vi "Post processing inversion hatch detector.vi"(7 "error in":errorcluster) -> (27 "error out":errorcluster)   [LabVIEW 2018]
uses:
  <vilib>/vision/NI_Vision_Development_Module.lvlib
panel:
  out "Particle Reports (Pixels)":T1(array[cluster]) {"Orientation" format="%.2f"; "Dimensions"."Height" format="%.2f"; "Dimensions"."Width" format="%.2f"; "Center of Mass"."Y" format="%.2f"; "Center of Mass"."X" format="%.2f"; "Bounding Rect"."Bottom" format="%.2f"; "Bounding Rect"."Right" format="%.2f"; "Bounding Rect"."Top" format="%.2f"; "Bounding Rect"."Left" format="%.2f"; "Number of Holes" format="%.2f"; "Area" format="%.2f"}
  out "Image Out 2":T2(plugin-control)
  in  "error in 2":errorcluster
  out "Image Out":T2(plugin-control)
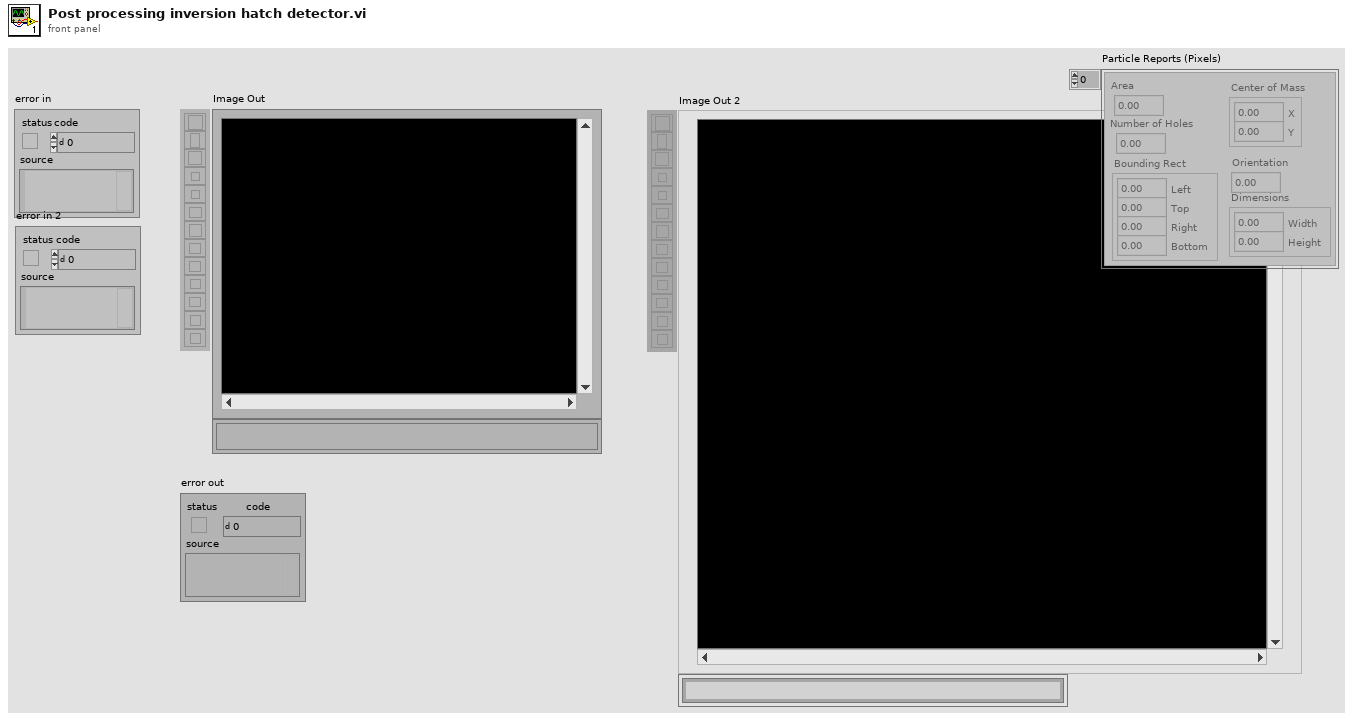
[diagram p1: front panel]
types:
  T1 = cluster{"Area":dbl, "Number of Holes":dbl, "Bounding Rect":cluster{"Left":dbl, "Top":dbl, "Right":dbl, "Bottom":dbl}, "Center of Mass":cluster{"X":dbl, "Y":dbl}, "Orientation":dbl, "Dimensions":cluster{"Width":dbl, "Height":dbl}}[]
  T2 = typedef "IMAQ Image.ctl" = refnum<image>
  T3 = cluster{"Desired Font (Application)":enum16{"User-specified Font", "Application Font", "System Font", "Dialog Font"}, "[User-specified Font]":cluster{"Font Name":string, "Size":i16, "Strikeout?":bool, "Italic?":bool, "Underline?":bool, "Outline?":bool, "Shadow?":bool, "Bold?":bool, "Rotation Angle":dbl}, "Horizontal Alignment":i16, "Vertical Alignment":i16}
  T4 = typedef "Image Type" = u32
  T5 = cluster{"Measurement Parameter":i32, "Range Lower Value":dbl, "Range Upper Value":dbl, "Range":bool, "Measurement Type":bool}[]
  T6 = cluster{"Area":dbl, "Number of Holes":dbl, "Bounding Rect":cluster{"Left":dbl, "Top":dbl, "Right":dbl, "Bottom":dbl}, "Center of Mass":cluster{"X":dbl, "Y":dbl}, "Orientation":dbl, "Dimensions":cluster{"Width":dbl, "Height":dbl}}
  T7 = cluster{"Left":dbl, "Top":dbl, "Right":dbl, "Bottom":dbl}
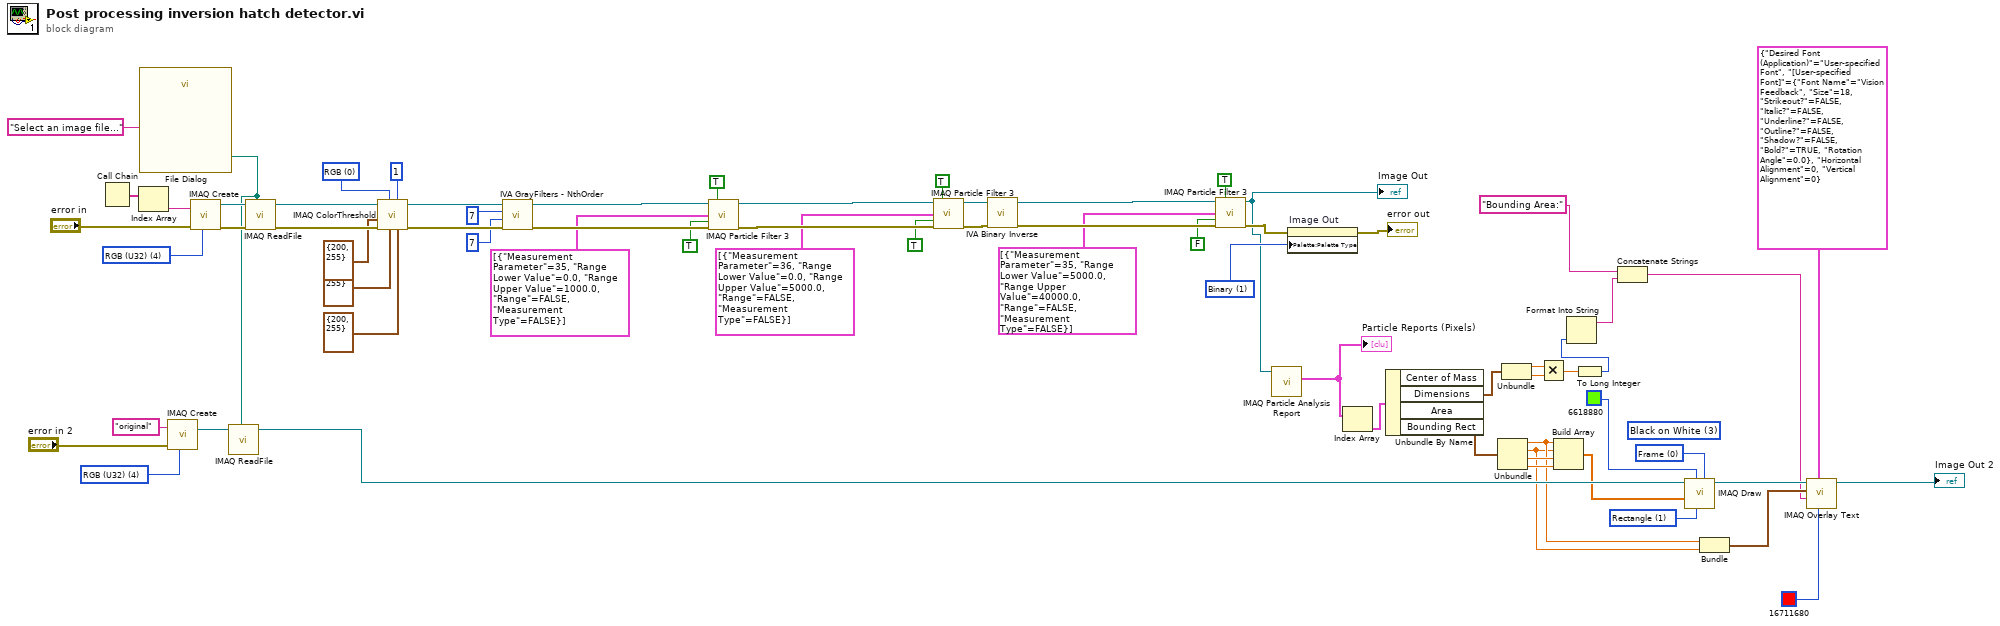
[diagram p0: block diagram]
diagram:
  (unwired) 3 items=["White", "Black", "Inverted", "Black on White", "White on Black"] ("Color")
  w21 = u16 1 items=["Line", "Rectangle", "Oval"] ("Shape to draw")
  w22 = u16 0 items=["Frame", "Paint", "Invert Frame", "Invert Paint"] ("Draw Mode")
  w31 = T4 4 items=["Grayscale (U8)", "Grayscale (I16)", "Grayscale (SGL)", "Complex (CSG)", "RGB (U32)", "HSL (U32)", "RGB (U64)", "Grayscale (U16)"] ("Image Type")
  w32 = u32 1 items=["Grayscale", "Binary", "Gradient", "Rainbow", "Temperature", "User Defined", "Binary 16 Bit", "Gradient 16 Bit", "Rainbow 16 Bit", "Temperature 16 Bit", "User Defined 16 Bit"] ("Palette Type")
  w60 = u16 0 items=["RGB", "HSL", "HSV", "HSI"] ("Color Mode")
  w62 = T4 4 items=["Grayscale (U8)", "Grayscale (I16)", "Grayscale (SGL)", "Complex (CSG)", "RGB (U32)", "HSL (U32)", "RGB (U64)", "Grayscale (U16)"] ("Image Type")
  n1 = Call Chain() -> (call chain=w65:string[])
  n2 = Index Array(array=w65) -> (element=w64:string)  [unwired: 1 in]
  n3 = call "File Dialog"("prompt"="Select an image file...") -> ("selected path"=w27:path)  [unwired: 6 in, 8 out]
  n4 = call "IMAQ Create"("Image Name"="original", "Image Type"=w31, "error in (no error)"="error in 2") -> ("New Image"=w28:T2)  [unwired: 1 in, 2 out]
  n5 = call "IMAQ Create"("Image Name"=w64, "Image Type"=w62, "error in (no error)"="error in") -> ("New Image"=w68:T2, "error out"=w67:errorcluster)  [unwired: 1 in, 1 out]
  n6 = call "IMAQ ReadFile"("File Path"=w27, "Image"=w28) -> ("Image Out"=w23:T2)  [unwired: 3 in, 6 out]
  n7 = call "IMAQ ReadFile"("File Path"=w27, "error in (no error)"=w67, "Image"=w68) -> ("error out"=w69:errorcluster, "Image Out"=w56:T2)  [unwired: 2 in, 5 out]
  n8 = call "IMAQ ColorThreshold"("Blue or Luma or Val or Inten Range"=cluster{"Lower value":i32, "Upper value":i32} {"Lower value"=200, "Upper value"=255}, "Replace Value"=1, "Green or Sat Range"=cluster{"Lower value":i32, "Upper value":i32} {"Lower value"=200, "Upper value"=255}, "Color Mode"=w60, "error in (no error)"=w69, "Red or Hue Range"=cluster{"Lower value":i32, "Upper value":i32} {"Lower value"=200, "Upper value"=255}, "Image Src"=w56) -> ("error out"=w55:errorcluster, "Image Dst Out"=w54:T2)  [unwired: 1 in, 2 out]
  n9 = call <vilib>:"IVA GrayFilters - NthOrder.vi"("error in"=w55, "Filter size Y"=7, "Filter size X"=7, "Image In"=w54) -> ("error out"=w53:errorcluster, "Image Out"=w47:T2)  [unwired: 6 out]
  n10 = call "IMAQ Particle Filter 3"("Image Src"=w47, "Connectivity 4/8 (8)"=TRUE, "Selection Values"=T5 [{"Measurement Parameter"=35, "Range Lower Value"=0.0, "Range Upper Value"=1000.0, "Range"=FALSE, "Measurement Type"=FALSE}], "Keep/Remove Particles (F)"=TRUE ("Keep/Remove Particles"), "error in (no error)"=w53) -> ("Image Dst Out"=w42:T2, "error out"=w48:errorcluster)  [unwired: 4 in, 5 out]
  n11 = call "IMAQ Particle Filter 3"("Image Src"=w42, "Connectivity 4/8 (8)"=TRUE, "Selection Values"=T5 [{"Measurement Parameter"=36, "Range Lower Value"=0.0, "Range Upper Value"=5000.0, "Range"=FALSE, "Measurement Type"=FALSE}], "Keep/Remove Particles (F)"=TRUE ("Keep/Remove Particles"), "error in (no error)"=w48) -> ("Image Dst Out"=w40:T2, "error out"=w43:errorcluster)  [unwired: 4 in, 5 out]
  n12 = call <vilib>:"IVA Binary Inverse.vi"("error in (no error)"=w43, "Image In"=w40) -> ("error out"=w39:errorcluster, "Image Out"=w35:T2)  [unwired: 8 out]
  n13 = call "IMAQ Particle Filter 3"("Image Src"=w35, "Connectivity 4/8 (8)"=TRUE, "Selection Values"=T5 [{"Measurement Parameter"=35, "Range Lower Value"=5000.0, "Range Upper Value"=40000.0, "Range"=FALSE, "Measurement Type"=FALSE}], "Keep/Remove Particles (F)"=FALSE ("Keep/Remove Particles"), "error in (no error)"=w39) -> ("Image Dst Out"=w26:T2, "error out"=w36:errorcluster)  [unwired: 4 in, 5 out]
  "Image Out" <- w26
  n14 = call "IMAQ Particle Analysis Report"("Image"=w26) -> ("Particle Reports (Pixels)"=w25:T1)  [unwired: 5 in, 5 out]
  "Particle Reports (Pixels)" <- w25
  n15 = property on="Image Out" class="ImageControl"(error in=w36, "Palette:Palette Type"=w32) -> (error out=→"error out":errorcluster)  [unwired: 1 in, 1 out]
  n16 = Index Array(array=w25) -> (element=w24:T6)  [unwired: 1 in]
  n17 = Unbundle By Name(w24) -> ("Dimensions"=w6:cluster{"Width":dbl, "Height":dbl}, "Bounding Rect"=w20:T7)  [unwired: 2 out]
  n18 = Unbundle(w20) -> ("Left"=w16:dbl, "Top"=w15:dbl, "Right"=w19:dbl, "Bottom"=w18:dbl)
  n19 = Unbundle(w6) -> ("Width"=w4:dbl, "Height"=w5:dbl)
  n20 = Multiply(x=w4, y=w5) -> (x*y=w2:dbl)
  n21 = Build Array(w16, w15, w19, w18) -> (w17:dbl[])
  n22 = To Long Integer(number=w2) -> (32bit integer=w1:i32)
  n23 = Format Into String(w1) -> (resulting string=w3:string)  [unwired: 3 in, 1 out]
  n24 = Concatenate Strings("Bounding Area:" ("string"), w3) -> (w11:string)
  n25 = call "IMAQ Draw"("Draw Mode"=w22, "Shape to draw"=w21, "Pixel Color"=u32 6618880, "Coordinates"=w17, "Image Src"=w23) -> ("Image Dst Out"=w12:T2)  [unwired: 5 in, 1 out]
  n26 = Bundle("Left"=w16, "Top"=w15) -> (w13:cluster{"Left":dbl, "Top":dbl})  [unwired: 1 in]
  n27 = call "IMAQ Overlay Text"("Text Color (black)"=u32 16711680, "Font, Size & Style"=T3 {"Desired Font (Application)"=enum."User-specified Font", "[User-specified Font]"={"Font Name"="Vision Feedback", "Size"=18, "Strikeout?"=FALSE, "Italic?"=FALSE, "Underline?"=FALSE, "Outline?"=FALSE, "Shadow?"=FALSE, "Bold?"=TRUE, "Rotation Angle"=0.0}, "Horizontal Alignment"=0, "Vertical Alignment"=0}, "String"=w11, "Origin"=w13, "Image"=w12) -> ("Image Out"=→"Image Out 2":T2)  [unwired: 5 in, 1 out]
